vi "GRBLCore.vi"(4 "SecondaryDataFeed":refnum<queue>, 5 "NumOfAxis":i32=3, 6 "MotorDisabled":refnum<vi>, 7 "Simulation":bool, 8 "error in":errorcluster, 9 "Serial Configuration":T2={"Baud Rate"=115200, "Parity"=0, "Data Bits"=8, "Stop Bits"=10, "Flow Control"=0} {"Flow Control" items=["None", "XON/XOFF", "RTS/CTS", "XON/XOFF & RTS/CTS", "DTR/DSR", "XON/XOFF & DTR/DSR"]; "Stop Bits" items=["1.0"=10, "1.5"=15, "2.0"=20]; "Data Bits" items=["7"=7, "8"=8]; "Parity" items=["None", "Odd", "Even", "Mark", "Space"]; "Baud Rate" items=["300"=300, "600"=600, "1200"=1200, "2400"=2400, "4800"=4800, "9600"=9600, "19200"=19200]}, 10 "CommPort":refnum<visa-resource-name>, 11 "ControlQueue in":refnum<queue>) -> (0 "error out":errorcluster, 3 "queue out":refnum<queue>)   [LabVIEW 2014, in "GRBLMotionCore.lvlib"]
uses:
  <instrlib>/GRBL/GRBLMotionCore.lvlib
  <instrlib>/GRBL/Public/Data/GRBL_State.ctl
  <instrlib>/GenericMotionCore/Public/SecondaryDataFeed.ctl
  <instrlib>/GRBL/Public/Data/GRBL_Data.ctl
  <vilib>/Utility/error.llb/DialogType.ctl
  <userlib>/Utility/ErrorLog_lib.lvlib
  <instrlib>/GenericMotionCore/GenericMotionCore.lvlib
panel:
  out "State(Blocking)":T1(ring)
  out "Blokcing Loop cts":i32
  in  "Track Input":bool
  in  "SoftReset":bool caption="Go"
  out "Com failure#":i32
  in  "Go_MoveRel":bool caption="Go"
  out "tick_start":u32
  out "tick_stop":u32
  out "Returned_String":string
  out "refresh rate":i32
  out "resfresh counter":i32
  in  "MotorDisabled":bool caption="Go"
  in  "Home":bool caption="Go"
  in  "StepWidth":dbl(ring)=0.2 items=["0.2 um"=0.0002, "0.001 mm"=0.001, "0.002 mm"=0.002, "0.005 mm "=0.005, "0.01 mm"=0.01, "0.02 mm"=0.02, "0.05 mm"=0.05, "0.1 mm"=0.1, "0.2 mm"=0.2, "1 mm"=1.0]
  in  "Z-":bool
  in  "Z+":bool
  in  "X+":bool
  in  "X-":bool
  in  "Y-":bool
  in  "Y+":bool
  in  "ClearErr":bool caption="Go"
  in  "STOP":bool caption="Go"
  in  "Quit":bool caption="Go"
  out "Instrument Driver Revision":string
  out "Instrument Firmware Revision":string
  in  "SetPosition":dbl[](array[numeric])=[1.0, 1.0, 1.0] caption="Position" format="%.4f"
  in  "SetVelocity":dbl[](array[numeric])=[1.0] caption="Velocity (mm/s)"
  in  "SetAcceleration":dbl[](array[numeric])=[50.0] caption="Acceleration"
  in  "Go":bool
  out "Moving":bool
  out "Acceleration":dbl[](array[numeric])
  out "Velocity":dbl[](array[numeric])
  out "Position":dbl[](array[numeric])
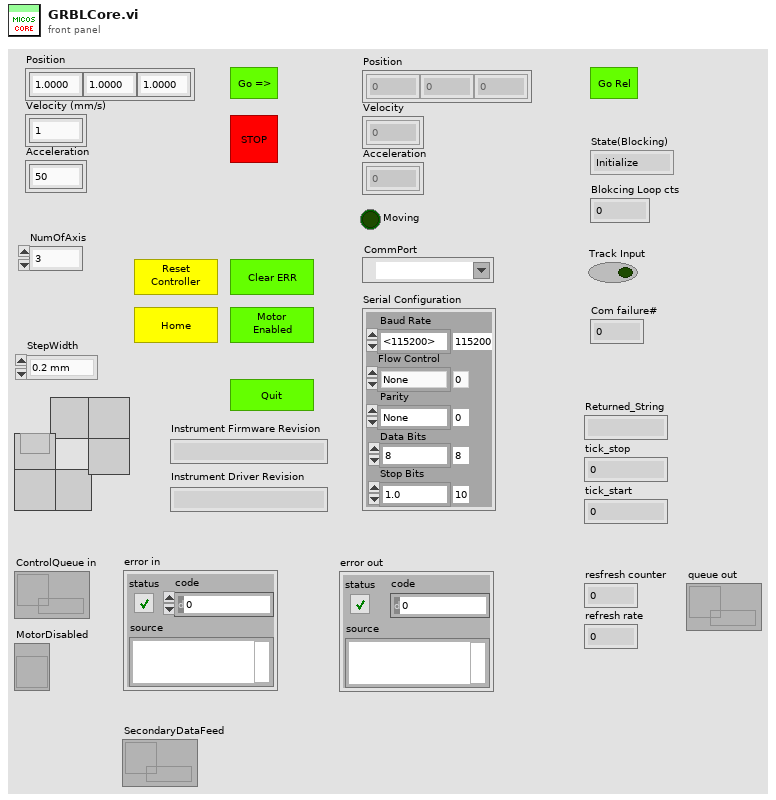
[diagram p1: front panel]
types:
  T1 = enum16{"Initialize", "SetDefaultConfig", "Close", "Quit", "Identify", "MoveAbs", "MoveAbs_all", "MoveRel", "MoveRel_all", "STOP", "Origin/Home", "WaitStop", "QueryStatus", "UpdateXPos", "UpdateAll", "SetVelocity", "SetAcceleration", "ClearErr", "LogMessage", "MotorEnable(1)", "EnableAxis", "JoyStick", "GetVelocity", "GetAcceleration", "SendCmd", "SetSoftLimits", "Beep", "_SettingReturn", "SoftReset"}
  T2 = cluster{"Baud Rate":u32, "Parity":u16, "Data Bits":u16, "Stop Bits":u16, "Flow Control":u16}
  T3 = cluster{"CommPort":refnum<vi>, "Serial Configuration":refnum<vi>, "SetPosition":refnum<vi>, "SetAcceleration":refnum<vi>, "SetVelocity":refnum<vi>, "StepWidth":refnum<vi>, "WaitStopReturn_Queue":refnum<queue>}
  T4 = typedef "GRBLMotionCore.lvlib/GRBL_State.ctl" = cluster{"State":enum16{"Initialize", "SetDefaultConfig", "Close", "Quit", "Identify", "MoveAbs", "MoveAbs_all", "MoveRel", "MoveRel_all", "STOP", "Origin/Home", "WaitStop", "QueryStatus", "UpdateXPos", "UpdateAll", "SetVelocity", "SetAcceleration", "ClearErr", "LogMessage", "MotorEnable(1)", "EnableAxis", "JoyStick", "GetVelocity", "GetAcceleration", "SendCmd", "SetSoftLimits", "Beep", "_SettingReturn", "SoftReset"}, "Params.":variant}
  T5 = typedef "GRBLMotionCore.lvlib/GRBL_Data.ctl" = cluster{"Position":dbl[], "Velocity":dbl[], "Acceleration":dbl[], "Moving":bool, "Simulation":bool, "tickcount_mov":u32, "tickcount_pos":u32, "NumOfAxis":i32, "Initialized":bool, "CommPort":refnum<visa-resource-name>, "Range":dbl[][], "Serial Configuration":cluster{"Baud Rate":u32, "Parity":u16, "Data Bits":u16, "Stop Bits":u16, "Flow Control":u16}, "MotorDisabled":refnum<vi>}
  T6 = typedef "StepWidthSelector.ctl" = dbl
  T7 = typedef "GenericMotionCore.lvlib/SecondaryDataFeed.ctl" = cluster{"tickcount":u32, "SecondaryData":dbl[]}
  T8 = enum16{"Initialize", "SetDefaultConfig", "Close", "Quit", "Identify", "MoveAbs", "MoveAbs_all", "MoveRel", "MoveRel_all", "STOP", "Origin/Home", "WaitStop", "QueryStatus", "UpdateXPos", "UpdateAll", "SetVelocity", "SetAcceleration", "ClearErr", "LogMessage", "MotorEnable(1)", "EnableAxis", "JoyStick", "GetVelocity", "GetAcceleration", "SendCmd", "SetSoftLimits", "Beep", "_SettingReturn"}
  T9 = enum16{"Initialize", "SetDefaultConfig", "Close", "Quit", "Identify", "MoveAbs", "MoveAbs_all", "MoveRel", "MoveRel_all", "STOP", "Origin/Home", "WaitStop", "QueryStatus", "UpdateXPos", "UpdateAll", "SetVelocity", "SetAcceleration", "ClearErr", "LogMessage", "MotorEnable(1)", "EnableAxis", "JoyStick", "GetVelocity", "GetAcceleration", "SendCmd", "SetSoftLimits", "Beep", "_SettingReturn"}[]
  T10 = typedef "DialogType.ctl" = u16
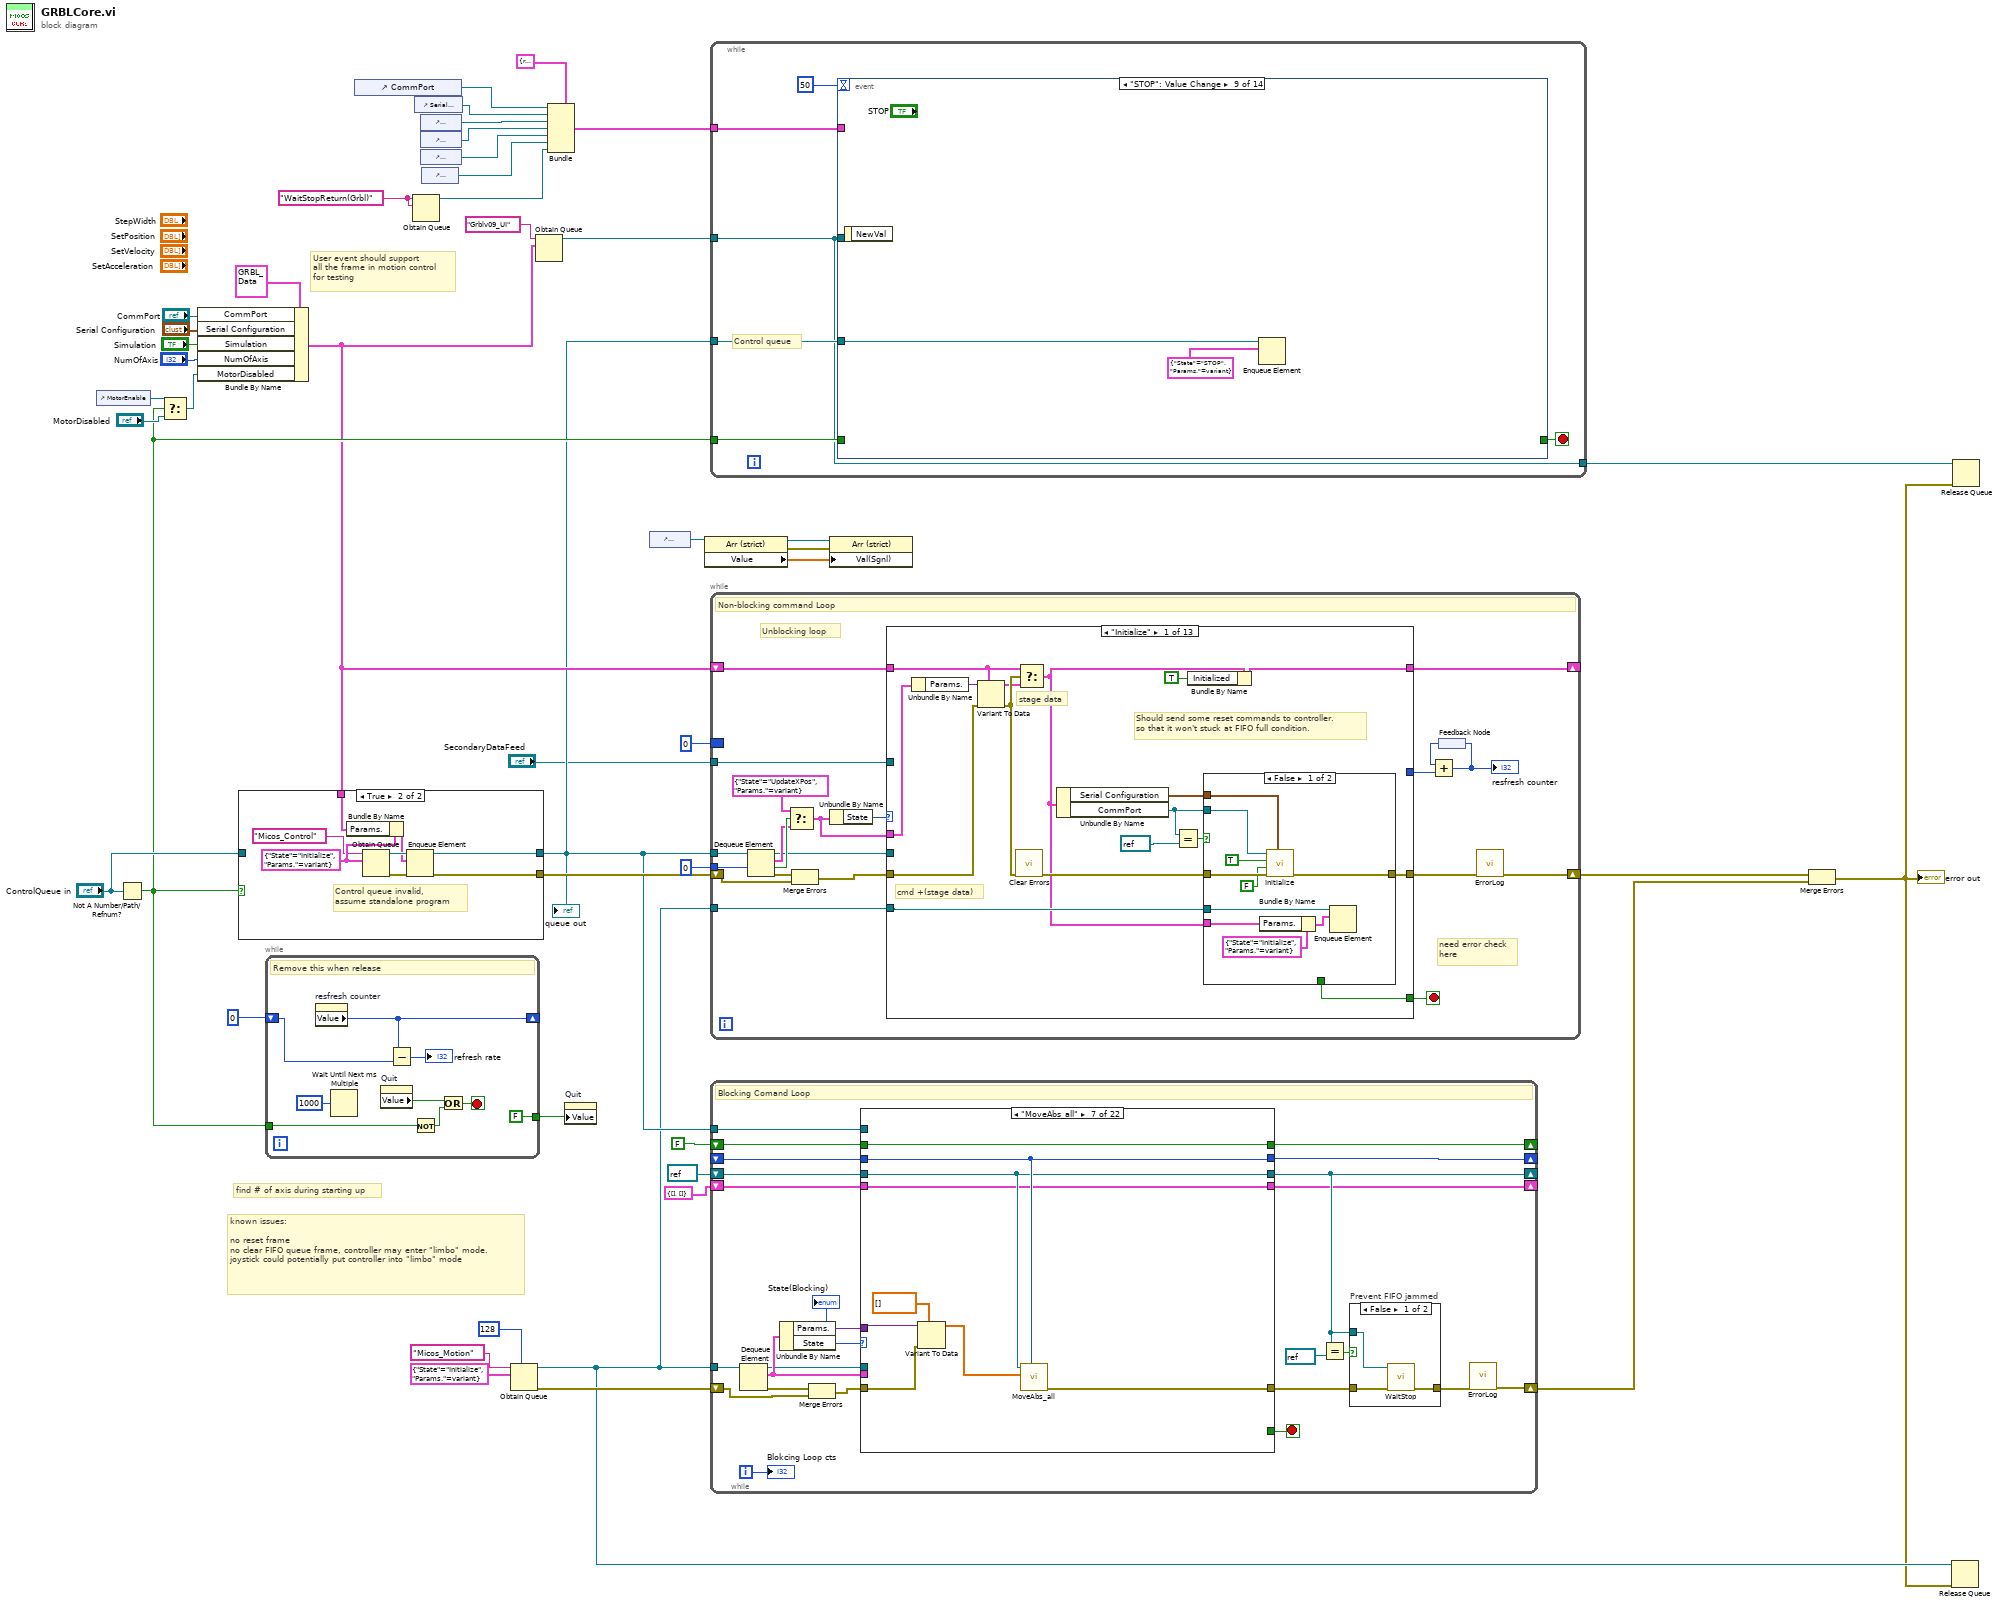
[diagram p0: block diagram]
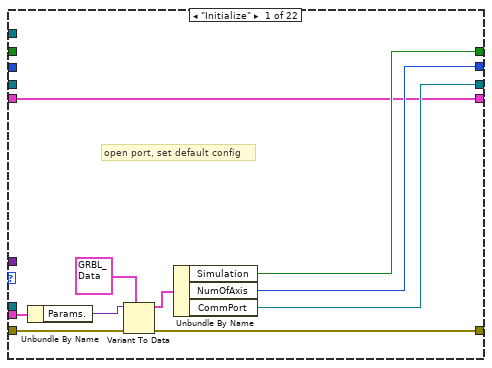
[diagram p3: hidden frame]
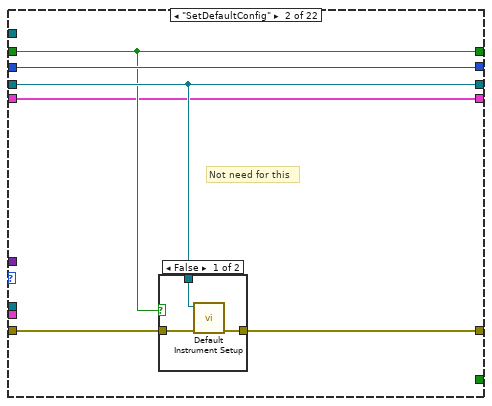
[diagram p4: hidden frame]
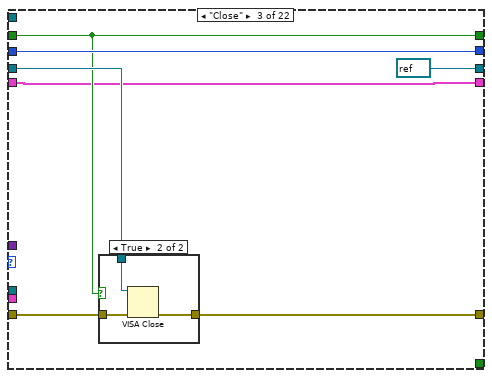
[diagram p6: hidden frame]
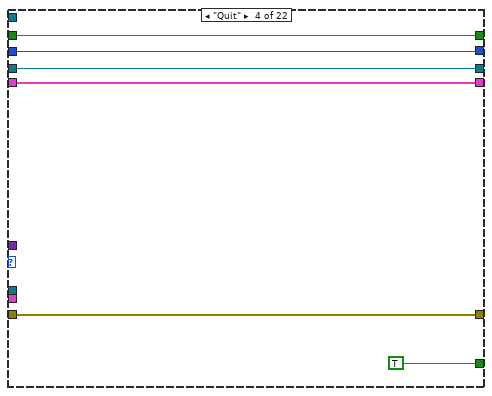
[diagram p8: hidden frame]
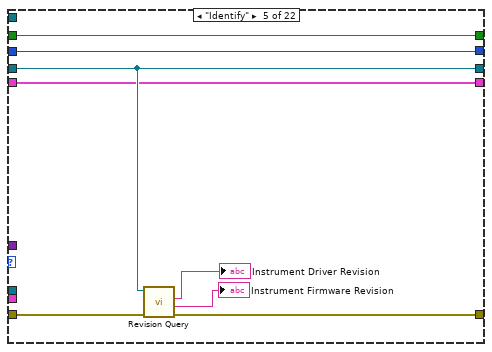
[diagram p9: hidden frame]
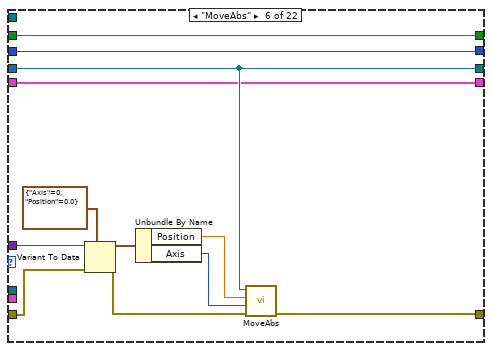
[diagram p10: hidden frame]
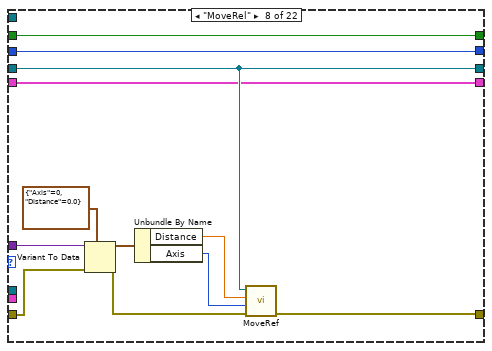
[diagram p11: hidden frame]
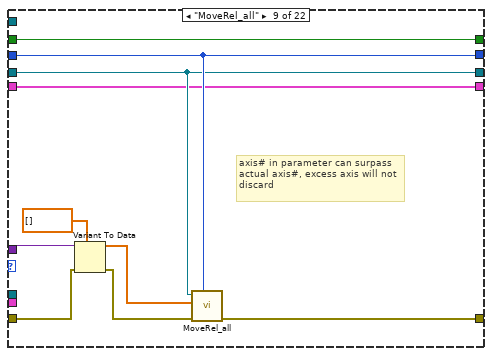
[diagram p12: hidden frame]
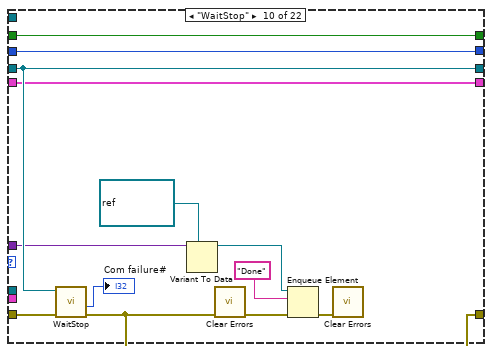
[diagram p13: hidden frame]
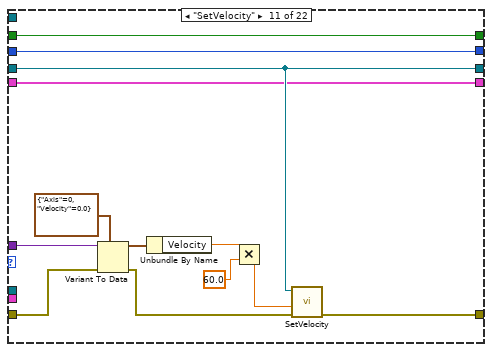
[diagram p14: hidden frame]
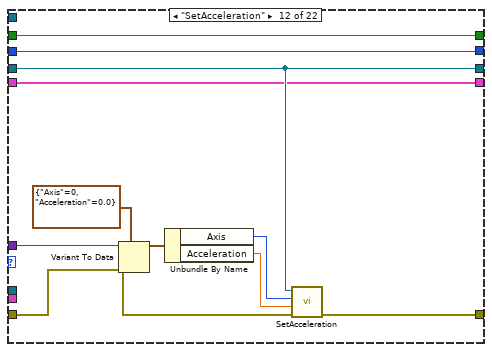
[diagram p15: hidden frame]
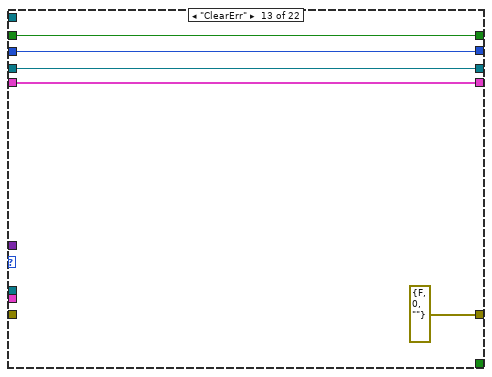
[diagram p16: hidden frame]
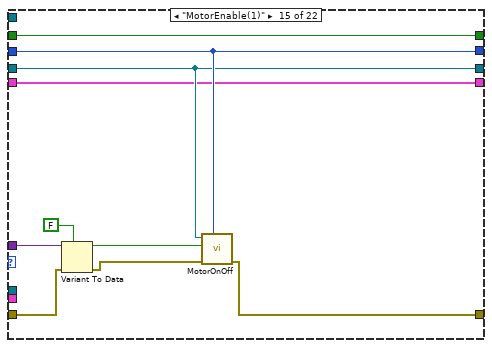
[diagram p18: hidden frame]
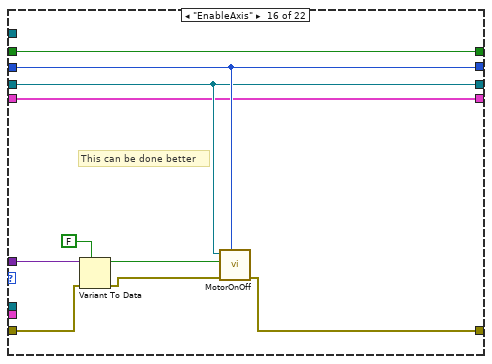
[diagram p19: hidden frame]
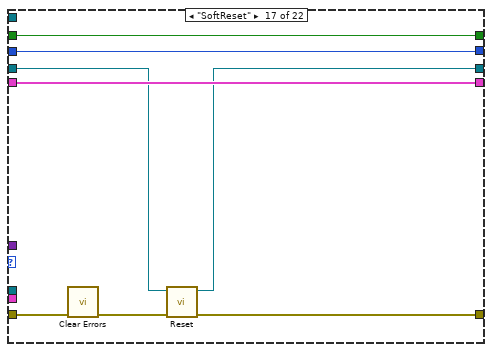
[diagram p20: hidden frame]
diagram:
  w21 = "WaitStopReturn(Grbl)" ("name (unnamed)")
  # "known issues:\n\nno reset frame\nno clear FIFO queue frame, controller may enter \"limbo\" mode. \njoystick could potentially put controller into \"limbo\" mode"
  # "find # of axis during starting up"
  # "User event should support \nall the frame in motion control\nfor testing"
  n1 = control-ref of="MotorEnable"() -> (w28:refnum<vi>)
  n2 = Not A Number/Path/Refnum?(number/path/refnum="ControlQueue in") -> (NaN/Path/Refnum?=w23:bool)
  n3 = Select(t=w28, s=w23, f="MotorDisabled") -> (s? t:f=w26:refnum<vi>)
  n4 = Bundle By Name(cluster=T5 {"Position"=[], "Velocity"=[], "Acceleration"=[], "Moving"=FALSE, "Simulation"=FALSE, "tickcount_mov"=0, "tickcount_pos"=0, "NumOfAxis"=0, "Initialized"=FALSE, "CommPort"="", "Range"=[], "Serial Configuration"={"Baud Rate"=0, "Parity"=0, "Data Bits"=0, "Stop Bits"=0, "Flow Control"=0}, "MotorDisabled"=refnum}, "CommPort"="CommPort", "Serial Configuration"="Serial Configuration", "Simulation"="Simulation", "NumOfAxis"="NumOfAxis", "MotorDisabled"=w26) -> (w22:T5)
  n5 = case shown="True" w23 {
    tunnel: [w48 w54] -> w17
    tunnel: ["error in" w53] -> w46
    tunnel: "ControlQueue in" -> [w48 _]
    tunnel: w22 -> [_ w50]
    frame False {
    }
    frame True {
      w55 = T4 {"State"=enum."Initialize", "Params."=variant}
      # "Control queue invalid, \nassume standalone program"
      n6 = Bundle By Name(cluster=w55, "Params."=w50) -> (w51:T4)
      n7 = Obtain Queue(name (unnamed)="Micos_Control", element data type=w55) -> (queue out=w56:refnum<queue>, error out=w52:errorcluster)  [unwired: 3 in, 1 out]
      n8 = Enqueue Element(queue=w56, element=w51, error in (no error)=w52) -> (queue out=w54:refnum<queue>, error out=w53:errorcluster)  [unwired: 1 in, 1 out]
    }
  }
  "queue out" <- w17
  n9 = while {
    shift-right: [w62] -> _
    shift-left: 0 ("resfresh counter") -> [w65]
    tunnel: w23 -> [w59]
    tunnel: [FALSE ("Quit")] -> w5
    stop <- w60 stop-if-true
    # "Remove this when release"
    n10 = property on="resfresh counter" class="DigNum (strict)"() -> ("Value"=w62:i32)  [unwired: 2 in, 2 out]
    n11 = Wait Until Next ms Multiple(millisecond multiple=u32 1000) -> ()  [unwired: 1 out]
    n12 = property on="Quit" class="Bool (strict)"() -> ("Value"=w63:bool)  [unwired: 2 in, 2 out]
    n13 = Subtract(x=w62, y=w65) -> (x-y=→"refresh rate":i32)
    n14 = Not(x=w59) -> (.not. x?=w58:bool)
    n15 = Or(x=w63, y=w58) -> (x .or. y?=w60:bool)
  }
  n16 = control-ref of="CommPort"() -> (w38:refnum<vi>)
  n17 = Obtain Queue(name (unnamed)=w21, element data type=w21) -> (queue out=w20:refnum<queue>)  [unwired: 3 in, 2 out]
  n18 = control-ref of="Serial Configuration"() -> (w39:refnum<vi>)
  n19 = control-ref of="SetPosition"() -> (w37:refnum<vi>)
  n20 = control-ref of="SetAcceleration"() -> (w36:refnum<vi>)
  n21 = control-ref of="SetVelocity"() -> (w35:refnum<vi>)
  n22 = control-ref of="StepWidth"() -> (w29:refnum<vi>)
  n23 = Obtain Queue(max queue size (-1, unlimited)=128, name (unnamed)="Micos_Motion", element data type=T4 {"State"=enum."Initialize", "Params."=variant}) -> (queue out=w15:refnum<queue>, error out=w43:errorcluster)  [unwired: 2 in, 1 out]
  n24 = Obtain Queue(name (unnamed)="Grblv09_UI", element data type=w22) -> (queue out=w18:refnum<queue>)  [unwired: 3 in, 2 out]
  n25 = Bundle(cluster=T3 {"CommPort"=refnum, "Serial Configuration"=refnum, "SetPosition"=refnum, "SetAcceleration"=refnum, "SetVelocity"=refnum, "StepWidth"=refnum, "WaitStopReturn_Queue"=refnum}, "CommPort"=w38, "Serial Configuration"=w39, "SetPosition"=w37, "SetAcceleration"=w36, "SetVelocity"=w35, "StepWidth"=w29, "WaitStopReturn_Queue"=w20) -> (w34:T3)
  n26 = property on="Quit" class="Bool (strict)"("Value"=w5) -> ()  [unwired: 2 in, 2 out]
  n27 = control-ref of="SetVelocity"() -> (w1:refnum<vi>)
  n28 = property class="Arr (strict)"(reference=w1) -> (reference out=w2:refnum<vi>, error out=w3:errorcluster, "Value"=w4:dbl[])  [unwired: 1 in]
  n29 = while {
    tunnel: w17 -> [w67]
    tunnel: w23 -> [w70]
    tunnel: w18 -> [w66]
    tunnel: w34 -> [w68]
    tunnel: [w66] -> w16
    stop <- w71 stop-if-true
    # "Control queue"
    n30 = event shown="[8] \"STOP\": Value Change" {
      selector: _ -> [_ _ _ _ _ _ _ _ _ _ _ _ _ _]
      dyn-events: _ -> [_ _ _ _ _ _ _ _ _ _ _ _ _ _]
      timeout: 50 -> [_ _ _ _ _ _ _ _ _ _ _ _ _ _]
      tunnel: [w74 _ _ _ _ _ _ _ _ _ _ TRUE _ _] -> w71
      tunnel: w70 -> [w87 _ _ _ _ _ _ _ _ _ _ _ _ _]
      tunnel: w67 -> [w86 w106 w117 w126 w135 w146 _ w180 w186 w188 w193 w196 w199 w201]
      tunnel: w66 -> [w79 _ _ _ _ _ _ _ _ _ _ _ _ _]
      tunnel: w68 -> [w78 w105 w116 _ _ _ w158 w179 _ _ _ _ _ _]
      event Timeout {
        # "Send return queue ref"
        n31 = event-data() -> ()  [unwired: 1 in, 1 out]
        n32 = Unbundle By Name(w78) -> ("WaitStopReturn_Queue"=w73:refnum<queue>)
        n33 = Not(x=w87) -> (.not. x?=w74:bool)
        n34 = Bundle By Name(cluster=T4 {"State"=enum."QueryStatus", "Params."=variant} ("element"), "Params."=w79) -> (w84:T4)
        n35 = Enqueue Element(queue=w86, element=w84) -> (error out=w82:errorcluster)  [unwired: 2 in, 2 out]
        n36 = Dequeue Element(queue=w79, timeout in ms (-1)=1000, error in (no error)=w82) -> (element=w80:T5, timed out?=w81:bool)  [unwired: 2 out]
        n37 = case shown="False" w81 {
          tunnel: w80 -> [w95 _]
          frame False {
            n38 = Unbundle By Name(w95) -> ("Position"=→"Position":dbl[], "Velocity"=→"Velocity":dbl[], "Acceleration"=→"Acceleration":dbl[], "Moving"=→"Moving":bool)
          }
          frame True {
          }
        }
        n39 = Dequeue Element(queue=w73, timeout in ms (-1)=0) -> (queue out=w72:refnum<queue>, element=w77:string, timed out?=w76:bool)  [unwired: 1 in, 1 out]
        n40 = case "Non-blocking WaitStop in UI for testing" shown="False" w76 {
          tunnel: w77 -> [w89 _]
          frame False {
            # "Non-blocking Wait for testing"
            n41 = Tick Count (ms)() -> (millisecond timer value=→"tick_stop":u32)
            "Returned_String" <- w89
          }
          frame True {
          }
        }
        n42 = case "Release feedback queue if no UI" shown="True" w74 {
          tunnel: w72 -> [_ w88]
          frame False {
          }
          frame True {
            n43 = Release Queue(queue=w88) -> ()  [unwired: 2 in, 3 out]
          }
        }
      }
      event "Go": Value Change {
        n44 = Unbundle By Name(w105) -> ("WaitStopReturn_Queue"=w100:refnum<queue>, "SetPosition"=w104:refnum<vi>)
        n45 = event-data() -> ()  [unwired: 1 in, 1 out]
        n46 = flat-sequence {
          tunnel: w106 -> [w113]
          tunnel: w103 -> [w110]
          tunnel: [w109] -> w102
          tunnel: [w108] -> w101
          frame #0 {
            n47 = Tick Count (ms)() -> (millisecond timer value=→"tick_start":u32)
            n48 = Bundle By Name(cluster=T4 {"State"=enum."MoveAbs_all", "Params."=variant} ("element"), "Params."=w110) -> (w111:T4)
            n49 = Enqueue Element(queue=w113, element=w111) -> (queue out=w109:refnum<queue>, error out=w108:errorcluster)  [unwired: 2 in, 1 out]
          }
        }
        n50 = property class="Arr (strict)"(reference=w104) -> ("Value"=w103:dbl[])  [unwired: 1 in, 2 out]
        n51 = local write "Returned_String"("Done" ("Returned_String")) -> ()
        n52 = local write "tick_stop"(u32 0 ("tick_stop")) -> ()
        n53 = Bundle By Name(cluster=T4 {"State"=enum."WaitStop", "Params."=variant} ("element"), "Params."=w100) -> (w97:T4)
        n54 = Enqueue Element(queue=w102, element=w97, error in (no error)=w101) -> ()  [unwired: 1 in, 3 out]
      }
      event "Go_MoveRel": Value Change {
        n55 = event-data() -> ()  [unwired: 1 in, 1 out]
        n56 = Unbundle By Name(w116) -> ("SetPosition"=w115:refnum<vi>)
        n57 = flat-sequence {
          tunnel: w117 -> [w123]
          tunnel: w114 -> [w120]
          tunnel: [w119] -> _
          tunnel: [w118] -> _
          frame #0 {
            n58 = Bundle By Name(cluster=T4 {"State"=enum."MoveRel_all", "Params."=variant} ("element"), "Params."=w120) -> (w121:T4)
            n59 = Enqueue Element(queue=w123, element=w121) -> (queue out=w119:refnum<queue>, error out=w118:errorcluster)  [unwired: 2 in, 1 out]
          }
        }
        n60 = property class="Arr (strict)"(reference=w115) -> ("Value"=w114:dbl[])  [unwired: 1 in, 2 out]
      }
      event "SetPosition": Value Change {
        n61 = event-data() -> ("NewVal"=w125:dbl[])  [unwired: 1 in]
        n62 = case shown="True" "Track Input" {
          tunnel: w126 -> [_ w130]
          tunnel: w125 -> [_ w127]
          frame False {
          }
          frame True {
            n63 = Bundle By Name(cluster=T4 {"State"=enum."MoveAbs_all", "Params."=variant} ("element"), "Params."=w127) -> (w128:T4)
            n64 = Enqueue Element(queue=w130, element=w128) -> ()  [unwired: 2 in, 3 out]
          }
        }
      }
      event "SetVelocity": Value Change {
        n65 = event-data() -> ("NewVal"=w134:dbl[])  [unwired: 1 in]
        n66 = for {
          N: 1 -> [_]
          tunnel: w134 -> [w138] mode=indexing
          shift-right: [w137] -> w133
          shift-left: w135 -> [w137]
          i -> [w143]
          n67 = Increment(x=w143) -> (x+1=w142:i32)
          n68 = Bundle By Name(cluster=cluster{"Axis":i32, "Velocity":dbl} {"Axis"=0, "Velocity"=0.0}, "Velocity"=w138, "Axis"=w142) -> (w139:cluster{"Axis":i32, "Velocity":dbl})
          n69 = Bundle By Name(cluster=T4 {"State"=enum."SetVelocity", "Params."=variant} ("element"), "Params."=w139) -> (w141:T4)
          n70 = Enqueue Element(queue=w137, element=w141) -> ()  [unwired: 2 in, 3 out]
        }
        n71 = Enqueue Element(queue=w133, element=T4 {"State"=enum."GetVelocity", "Params."=variant}) -> ()  [unwired: 2 in, 3 out]
      }
      event "SetAcceleration": Value Change {
        n72 = event-data() -> ("NewVal"=w147:dbl[])  [unwired: 1 in]
        n73 = for {
          tunnel: w147 -> [w149] mode=indexing
          shift-right: [w148] -> w144
          shift-left: w146 -> [w148]
          i -> [w155]
          n74 = Increment(x=w155) -> (x+1=w153:i32)
          n75 = Bundle By Name(cluster=cluster{"Axis":i32, "Acceleration":dbl} {"Axis"=0, "Acceleration"=0.0}, "Acceleration"=w149, "Axis"=w153) -> (w150:cluster{"Axis":i32, "Acceleration":dbl})
          n76 = Bundle By Name(cluster=T4 {"State"=enum."SetAcceleration", "Params."=variant} ("element"), "Params."=w150) -> (w152:T4)
          n77 = Enqueue Element(queue=w148, element=w152) -> ()  [unwired: 2 in, 3 out]
        }
        n78 = Enqueue Element(queue=w144, element=T4 {"State"=enum."GetAcceleration", "Params."=variant}) -> ()  [unwired: 2 in, 3 out]
      }
      event "Position": Mouse Down {
        n79 = event-data() -> ("CtlRef"=w157:refnum<vi>, "Mods.Double Click"=w156:bool)  [unwired: 1 in]
        n80 = case shown="True" w156 {
          tunnel: w158 -> [_ w162]
          tunnel: w157 -> [_ w160]
          frame False {
          }
          frame True {
            n81 = Unbundle By Name(w162) -> ("SetPosition"=w161:refnum<vi>)
            n82 = property class="Arr (strict)"(reference=w160) -> ("Value"=w159:dbl[])  [unwired: 1 in, 2 out]
            n83 = property class="Arr (strict)"(reference=w161, "Value"=w159) -> ()  [unwired: 1 in, 2 out]
          }
        }
      }
      event "X+", "X-", "Y+", "Y-", "Z+", "Z-": Value Change {
        n84 = event-data() -> ()  [unwired: 1 in, 1 out]
        n85 = Unbundle By Name(w179) -> ("StepWidth"=w178:refnum<vi>)
        n86 = property class="Ring (strict)"(reference=w178) -> ("Value"=w170:T6)  [unwired: 1 in, 2 out]
        n87 = Build Array("X+", "X-", "Y+", "Y-", "Z+", "Z-") -> (w177:bool[])
        n88 = Search 1D Array(1D array=w177, element=TRUE) -> (index of element=w174:i32)  [unwired: 1 in]
        n89 = Index Array(array=dbl[] [1.0, -1.0, 1.0, -1.0, 1.0, -1.0], index=w174) -> (element=w173:dbl)
        n90 = Index Array(array=i32[] [1, 1, 2, 2, 3, 3], index=w174) -> (element=w169:i32)
        n91 = Multiply(x=w170, y=w173) -> (x*y=w171:T6)
        n92 = Bundle By Name(cluster=cluster{"Axis":i32, "Position":dbl} {"Axis"=0, "Position"=0.0}, "Position"=w171, "Axis"=w169) -> (w181:cluster{"Axis":i32, "Position":dbl})
        n93 = Bundle By Name(cluster=T4 {"State"=enum."MoveRel", "Params."=variant} ("element"), "Params."=w181) -> (w183:T4)
        n94 = Enqueue Element(queue=w180, element=w183) -> ()  [unwired: 2 in, 3 out]
      }
      event "STOP": Value Change {
        n95 = event-data() -> ()  [unwired: 1 in, 1 out]
        n96 = Enqueue Element(queue=w186, element=T4 {"State"=enum."STOP", "Params."=variant}) -> ()  [unwired: 2 in, 3 out]
      }
      event "Home": Value Change {
        n97 = event-data() -> ()  [unwired: 1 in, 1 out]
        n98 = Enqueue Element(queue=w188, element=T4 {"State"=enum."Origin/Home", "Params."=variant}) -> ()  [unwired: 2 in, 3 out]
      }
      event "MotorDisabled": Value Change {
        n99 = event-data() -> ()  [unwired: 1 in, 1 out]
        n100 = Not(x="MotorDisabled") -> (.not. x?=w189:bool)
        n101 = Bundle By Name(cluster=T4 {"State"=enum."MotorEnable(1)", "Params."=variant} ("element"), "Params."=w189) -> (w191:T4)
        n102 = Enqueue Element(queue=w193, element=w191) -> ()  [unwired: 2 in, 3 out]
      }
      event "Quit": Value Change {
        n103 = event-data() -> ()  [unwired: 1 in, 1 out]
        n104 = disable-structure shown="Disabled" {
          frame Disabled {
            n105 = property on="Quit" class="Bool (strict)"("Value"=FALSE ("Quit")) -> ()  [unwired: 2 in, 2 out]
          }
          frame Enabled {
          }
        }
        n106 = Enqueue Element(queue=w196, element=T4 {"State"=enum."Quit", "Params."=variant}) -> ()  [unwired: 2 in, 3 out]
      }
      event "ClearErr": Value Change {
        n107 = event-data() -> ()  [unwired: 1 in, 1 out]
        n108 = Enqueue Element(queue=w199, element=T4 {"State"=enum."ClearErr", "Params."=variant}) -> ()  [unwired: 2 in, 3 out]
      }
      event "SoftReset": Value Change {
        n109 = event-data() -> ()  [unwired: 1 in, 1 out]
        n110 = Enqueue Element(queue=w201, element=T4 {"State"=enum."SoftReset", "Params."=variant}) -> ()  [unwired: 2 in, 3 out]
      }
    }
  }
  n111 = while {
    tunnel: w17 -> [w212]
    shift-right: [w222] -> _
    shift-left: w22 -> [w221]
    tunnel: w15 -> [w219]
    shift-right: [w203] -> w8
    shift-left: w46 -> [w208]
    tunnel: 0 ("f") -> [w210]
    border: 0 -> [_]
    tunnel: "SecondaryDataFeed" -> [w202]
    stop <- w220 stop-if-true
    # "Unblocking loop"
    # "need error check\nhere"
    # "Non-blocking command Loop"
    n112 = Dequeue Element(queue=w212, timeout in ms (-1)=w210) -> (queue out=w213:refnum<queue>, element=w215:T4, timed out?=w217:bool, error out=w218:errorcluster)  [unwired: 1 in]
    n113 = Select(t=T4 {"State"=enum."UpdateXPos", "Params."=variant} ("element"), s=w217, f=w215) -> (s? t:f=w214:T4)
    n114 = Merge Errors(w218, w208) -> (w209:errorcluster)
    n115 = Unbundle By Name(w214) -> ("State"=w211:T1)
    n116 = case shown="\"Initialize\"" w211 {
      tunnel: w214 -> [w230 w262 _ _ w317 _ _ _ _ w429 w448 w460 w473]
      tunnel: [w239 w259 w279 w303 w313 w322 w345 w387 w425 w434 w451 w458 w475] -> w222
      tunnel: w221 -> [w233 w257 w279 w303 w313 w322 w343 w385 w425 w434 w451 w461 w475]
      tunnel: [w229 _ TRUE _ _ _ _ _ _ _ _ _ _] -> w220
      tunnel: w219 -> [w224 w263 w282 w302 _ _ _ w374 _ w433 w450 _ _]
      tunnel: [w232 w260 w284 w298 w315 w320 w336 w377 errorcluster {"status"=FALSE, "code"=0, "source"=""} ("error out") w426 w447 w452 w476] -> w204
      tunnel: w209 -> [w236 w261 w280 w301 w316 w323 w344 w386 _ w432 w449 w453 _]
      tunnel: w213 -> [_ w255 _ _ _ _ w335 _ _ w430 _ _ w468]
      tunnel: [_ _ _ _ _ _ 1 1 _ _ _ _ _] -> w207
      tunnel: w202 -> [_ _ _ _ _ _ w325 w371 _ _ _ _ _]
      frame "Initialize" {
        # "Should send some reset commands to controller. \nso that it won't stuck at FIFO full condition."
        # "cmd +(stage data)"
        # "stage data"
        n117 = Unbundle By Name(w230) -> ("Params."=w237:variant)
        n118 = Variant To Data(error in=w236, type=w233, Variant=w237) -> (data=w234:T5, error out=w235:errorcluster)
        n119 = call <vilib>:"Clear Errors.vi"("error in (no error)"=w235) -> ("error out"=w225:errorcluster)  [unwired: 5 in, 1 out]
        n120 = Select(t=w233, s=w235, f=w234) -> (s? t:f=w223:T5)
        n121 = Unbundle By Name(w223) -> ("Serial Configuration"=w231:T2, "CommPort"=w227:refnum<visa-resource-name>)
        n122 = Equal?(x=w227, y=refnum<visa-resource-name> refnum ("CommPort")) -> (x = y?=w228:bool)
        n123 = Bundle By Name(cluster=w223, "Initialized"=TRUE) -> (w239:T5)
        n124 = case shown="False" w228 {
          tunnel: w225 -> [w249 w252]
          tunnel: [w248 errorcluster {"status"=FALSE, "code"=-5104, "source"="Device unspecifiied,\nSkip execution"} ("error out")] -> w232
          tunnel: w231 -> [w247 _]
          tunnel: w227 -> [w246 _]
          tunnel: [_ w250] -> w229
          tunnel: w224 -> [w241 w254]
          tunnel: w223 -> [w240 _]
          frame False {
            n125 = Bundle By Name(cluster=T4 {"State"=enum."Initialize", "Params."=variant}, "Params."=w240) -> (w243:T4)
            n126 = call <instrlib>:"Initialize.vi"("Serial Configuration"=w247, "error in (no error)"=w249, "Reset (True)"=FALSE, "ID Query (True)"=TRUE, "VISA resource name"=w246) -> ("error out"=w248:errorcluster)  [unwired: 5 in, 1 out]
            n127 = Enqueue Element(queue=w241, element=w243) -> ()  [unwired: 2 in, 3 out]
          }
          frame True {
            w250 = TRUE
            n128 = Enqueue Element(queue=w254, element=T4 {"State"=enum."Quit", "Params."=variant}, error in (no error)=w252) -> ()  [unwired: 1 in, 3 out]
            n129 = property on="Quit" class="Bool (strict)"("Val(Sgnl)"=w250) -> ()  [unwired: 2 in, 2 out]
          }
        }
      }
      frame "Close" {
        n130 = Unbundle By Name(w257) -> ("Moving"=w256:bool)
        n131 = case shown="True" w256 {
          tunnel: w263 -> [w267 _]
          tunnel: w262 -> [w266 w268]
          tunnel: w261 -> [w265 w272]
          tunnel: [w264 w269] -> w260
          tunnel: w255 -> [_ w277]
          frame False {
            n132 = Enqueue Element "Imply \"Close\""(queue=w267, element=w266, error in (no error)=w265) -> (error out=w264:errorcluster)  [unwired: 1 in, 2 out]
          }
          frame True {
            n133 = Enqueue Element At Opposite End "Implied \"Close\""(queue=w277, element=w268, error in (no error)=w272) -> (queue out=w276:refnum<queue>, error out=w271:errorcluster)  [unwired: 1 in, 1 out]
            n134 = Enqueue Element At Opposite End(queue=w276, element=T4 {"State"=enum."UpdateAll", "Params."=variant}, error in (no error)=w271) -> (queue out=w275:refnum<queue>, error out=w270:errorcluster)  [unwired: 1 in, 1 out]
            n135 = Enqueue Element At Opposite End(queue=w275, element=T4 {"State"=enum."STOP", "Params."=variant}, error in (no error)=w270) -> (error out=w269:errorcluster)  [unwired: 1 in, 2 out]
          }
        }
        n136 = Bundle By Name(cluster=w257, "Initialized"=FALSE) -> (w259:T5)
      }
      frame "Quit" {
        n137 = Unbundle By Name(w279) -> ("Initialized"=w278:bool)
        n138 = case shown="True" w278 {
          tunnel: [w288 w292] -> w283
          tunnel: w282 -> [w288 w291]
          tunnel: [w287 w290] -> w281
          tunnel: w280 -> [w287 w289]
          frame False {
          }
          frame True {
            n139 = Enqueue Element(queue=w291, element=T4 {"State"=enum."Close", "Params."=variant}, error in (no error)=w289) -> (queue out=w292:refnum<queue>, error out=w290:errorcluster)  [unwired: 1 in, 1 out]
          }
        }
        n140 = Enqueue Element(queue=w283, element=T4 {"State"=enum."Quit", "Params."=variant}, error in (no error)=w281) -> (error out=w284:errorcluster)  [unwired: 1 in, 2 out]
      }
      frame "STOP" {
        w294 = T9 [enum."WaitStop", enum."UpdateAll", enum."Close", enum."Quit", enum."SetVelocity"] items=["Initialize", "SetDefaultConfig", "Close", "Quit", "Identify", "MoveAbs", "MoveAbs_all", "MoveRel", "MoveRel_all", "STOP", "Origin/Home", "WaitStop", "QueryStatus", "UpdateXPos", "UpdateAll", "SetVelocity", "SetAcceleration", "ClearErr", "LogMessage", "MotorEnable(1)", "EnableAxis", "JoyStick", "GetVelocity", "GetAcceleration", "SendCmd", "SetSoftLimits", "Beep", "_SettingReturn"]
        # "should not dump wait for stop!!"
        # "send stop to controller, update"
        n141 = Unbundle By Name(w303) -> ("CommPort"=w300:refnum<visa-resource-name>)
        n142 = Flush Queue(queue=w302, error in (no error)=w301) -> (queue out=w295:refnum<queue>, remaining elements=w296:T4[], error out=w299:errorcluster)
        n143 = VISA Write(VISA resource name=w300, write buffer="!\r\n" ("Substring"), error in (no error)=w299) -> (error out=w298:errorcluster)  [unwired: 2 out]
        n144 = for {
          tunnel: w296 -> [w309] mode=indexing
          tunnel: w295 -> [w308]
          tunnel: w294 -> [w306]
          n145 = Unbundle By Name(w309) -> ("State"=w307:T1)
          n146 = Equal?(x=w307, y=w306) -> (x = y?=w304:bool[])
          n147 = Or Array Elements(Boolean array=w304) -> (logical OR=w305:bool)
          n148 = case shown="True" w305 {
            tunnel: w309 -> [_ w311]
            tunnel: w308 -> [_ w310]
            frame False {
            }
            frame True {
              n149 = Enqueue Element At Opposite End(queue=w310, element=w311) -> ()  [unwired: 2 in, 3 out]
            }
          }
        }
      }
      frame "QueryStatus" {
        # "return the value to queue"
        n150 = Unbundle By Name(w317) -> ("Params."=w319:variant)
        n151 = Variant To Data(error in=w316, type=refnum<queue> refnum ("queue out"), Variant=w319) -> (data=w314:refnum<queue>, error out=w318:errorcluster)
        n152 = Enqueue Element(queue=w314, element=w313, error in (no error)=w318) -> (error out=w315:errorcluster)  [unwired: 1 in, 2 out]
      }
      frame "Origin/Home" {
        # "The stage won't work, if not calibrated/homed,\nSo calibration has to be in the non-blocking loop\n\nAlso, during calibration, communication stop, causing error"
        n153 = Unbundle By Name(w322) -> ("CommPort"=w321:refnum<visa-resource-name>)
        n154 = call <instrlib>:"OriginSearch.vi"("error in"=w323, "VISA resource"=w321) -> ("error out"=w320:errorcluster)  [unwired: 9 in]
      }
      frame "UpdateXPos" {
        n155 = Unbundle By Name(w343) -> ("NumOfAxis"=w329:i32, "CommPort"=w331:refnum<visa-resource-name>)
        n156 = feedback #1(0) -> (w339:i32)
        n157 = Increment(x=w339) -> (x+1=w340:i32)
        n158 = Quotient & Remainder(x=w340, y=16) -> (x-y*floor(x/y)=w337:i32)  [unwired: 1 out]
        n159 = feedback-in #1(w337) -> ()
        n160 = Equal To 0?(x=w337) -> (x = 0?=w334:bool)
        n161 = call <instrlib>:"Update_xPos.vi"("NumOfAxis"=w329, "error in (no error)"=w344, "VISA resource name"=w331) -> ("error out"=w327:errorcluster, "x_Moving"=w332:bool, "Position"=w330:dbl[], "tickcount_pos"=w342:u32)  [unwired: 5 in]
        n162 = Compound Arithmetic op=OR(invert w332, w334) -> (w333:bool)
        n163 = case shown="No Error" w327 {
          selector: w327 -> [w352 w357]
          tunnel: [w354 w360] -> w345
          tunnel: w343 -> [w353 w360]
          tunnel: w342 -> [w347 _]
          tunnel: w330 -> [w346 _]
          tunnel: [w352 w356] -> w326
          tunnel: w325 -> [w348 _]
          frame No Error {
            n164 = Bundle(cluster=T7 {"tickcount"=0, "SecondaryData"=[]} ("SecondaryDataFeed"), "tickcount"=w347, "SecondaryData"=w346) -> (w349:T7)
            n165 = Bundle By Name(cluster=w353, "tickcount_pos"=w347, "Position"=w346) -> (w354:T5)
            n166 = Lossy Enqueue Element(queue=w348, element=w349) -> (error out=w350:errorcluster)  [unwired: 1 in, 3 out]
            n167 = call <vilib>:"Clear Errors.vi"("error in (no error)"=w350) -> ()  [unwired: 5 in, 2 out]
          }
          frame Error {
            w355 = T10 0 items=["no dialog", "OK message", "continue or stop message", "OK message + warnings", "continue/stop + warnings"] ("type of dialog (OK msg:1)")
            w358 = 1 items=["no exception", "cancel error on match", "set error on match"] ("[exception action] (none:0)")
            n168 = for {
              shift-right: [w364] -> w356
              shift-left: w357 -> [w365]
              tunnel: w358 -> [w363]
              tunnel: i32[] [85, -1073807252, 1, -1073807339] -> [w362] mode=indexing
              tunnel: w355 -> [w361]
              n169 = call <vilib>:"General Error Handler.vi"("type of dialog (OK msg:1)"=w361, "error in (no error)"=w365, "[exception action] (none:0)"=w363, "[exception code]"=w362) -> ("error out"=w364:errorcluster)  [unwired: 7 in, 4 out]
            }
          }
        }
        n170 = Wait Until Next ms Multiple(millisecond multiple=u32 40) -> ()  [unwired: 1 out]
        n171 = case shown="True" w333 {
          tunnel: [w366 w370] -> w336
          tunnel: w335 -> [_ w369]
          tunnel: w326 -> [w366 w367]
          frame False {
          }
          frame True {
            n172 = Enqueue Element At Opposite End(queue=w369, element=T4 {"State"=enum."UpdateAll", "Params."=variant}, error in (no error)=w367) -> (error out=w370:errorcluster)  [unwired: 1 in, 2 out]
          }
        }
      }
      frame "UpdateAll" {
        n173 = Unbundle By Name(w385) -> ("MotorDisabled"=w376:refnum<vi>, "NumOfAxis"=w384:i32, "CommPort"=w383:refnum<visa-resource-name>)
        n174 = call <instrlib>:"Update_all.vi"("# axis"=w384, "error in (no error)"=w386, "VISA resource name"=w383) -> ("error out"=w378:errorcluster, "Moving"=w379:bool, "Currrent postion"=w382:dbl[], "tickcount_pos"=w381:u32, "MotorDisabled"=w372:bool)  [unwired: 4 in]
        n175 = property class="Bool (strict)"(reference=w376, "Blinking"=w372, "Value"=w372) -> (error out=w375:errorcluster)  [unwired: 1 in, 1 out]
        n176 = case shown="No Error" w378 {
          selector: w378 -> [_ w415]
          tunnel: [w406 w418] -> w387
          tunnel: w385 -> [w405 w418]
          tunnel: w382 -> [w389 _]
          tunnel: w381 -> [w390 _]
          tunnel: w379 -> [w403 _]
          tunnel: [_ w414] -> w377
          tunnel: w374 -> [w404 _]
          tunnel: T4[] [{"State"=enum."GetVelocity", "Params."=variant}, {"State"=enum."_SettingReturn", "Params."=variant}] -> [w402 _]
          tunnel: w371 -> [w388 _]
          frame No Error {
            w394 = FALSE  # Bypass  continuous update
            n177 = Tick Count (ms)() -> (millisecond timer value=w400:u32)
            n178 = feedback #2() -> (w396:u32)  [unwired: 1 in]
            n179 = Subtract(x=w400, y=w396) -> (x-y=w399:u32)
            n180 = Greater?(x=u32 1000, y=w399) -> (0:w401:bool)
            n181 = Compound Arithmetic op=OR(w394, w403, w401) -> (w395:bool)
            n182 = Bundle By Name(cluster=w405, "tickcount_pos"=w390, "Position"=w389, "Moving"=w403) -> (w406:T5)
            n183 = case shown="False" w395 {
              tunnel: w404 -> [w409 _]
              tunnel: w402 -> [w408 _]
              tunnel: [w407 w412] -> w397
              tunnel: w396 -> [_ w412]
              frame False {
                n184 = for {
                  tunnel: w409 -> [w411]
                  tunnel: w408 -> [w410] mode=indexing
                  n185 = Enqueue Element(queue=w411, element=w410) -> ()  [unwired: 2 in, 3 out]
                }
                n186 = Tick Count (ms)() -> (millisecond timer value=w407:u32)
              }
              frame True {
              }
            }
            n187 = feedback-in #2(w397) -> ()
            n188 = Bundle(cluster=T7 {"tickcount"=0, "SecondaryData"=[]} ("SecondaryDataFeed"), "tickcount"=w390, "SecondaryData"=w389) -> (w391:T7)
            n189 = Lossy Enqueue Element(queue=w388, element=w391) -> (error out=w392:errorcluster)  [unwired: 1 in, 3 out]
            n190 = call <vilib>:"Clear Errors.vi"("error in (no error)"=w392) -> ()  [unwired: 5 in, 2 out]
          }
          frame Error {
            w413 = T10 0 items=["no dialog", "OK message", "continue or stop message", "OK message + warnings", "continue/stop + warnings"] ("type of dialog (OK msg:1)")
            w417 = 1 items=["no exception", "cancel error on match", "set error on match"] ("[exception action] (none:0)")
            n191 = for {
              shift-right: [w422] -> w414
              shift-left: w415 -> [w423]
              tunnel: w417 -> [w421]
              tunnel: i32[] [85, -1073807252, -1073807339, 1] -> [w420] mode=indexing
              tunnel: w413 -> [w419]
              n192 = call <vilib>:"General Error Handler.vi"("type of dialog (OK msg:1)"=w419, "error in (no error)"=w423, "[exception action] (none:0)"=w421, "[exception code]"=w420) -> ("error out"=w422:errorcluster)  [unwired: 7 in, 4 out]
            }
          }
        }
        n193 = call <vilib>:"Clear Errors.vi"("error in (no error)"=w375) -> ()  [unwired: 5 in, 2 out]
      }
      frame "ClearErr" {
      }
      frame Default {
        # "system does not response \nafter a command is received"
        # "timeout push command back then do update?\n\npreventing blocking"
        n194 = Enqueue Element(queue=w433, element=w429, timeout in ms (-1)=0, error in (no error)=w432) -> (timed out?=w427:bool, error out=w428:errorcluster)  [unwired: 1 out]
        n195 = case shown="True" w427 {
          tunnel: w430 -> [_ w443]
          tunnel: w429 -> [_ w442]
          tunnel: w428 -> [w435 w441]
          tunnel: [w435 w438] -> w426
          frame False {
          }
          frame True {
            w436 = 500  # Prevent core stuck, but cause loosing command
            n196 = Enqueue Element At Opposite End(queue=w443, element=w442, timeout in ms (-1)=w436, error in (no error)=w441) -> (queue out=w440:refnum<queue>, error out=w437:errorcluster)  [unwired: 1 out]
            n197 = Enqueue Element At Opposite End(queue=w440, element=T4 {"State"=enum."UpdateXPos", "Params."=variant}, timeout in ms (-1)=w436, error in (no error)=w437) -> (error out=w438:errorcluster)  [unwired: 2 out]
          }
        }
      }
      frame "GetVelocity", "GetAcceleration" {
        # "system does not response \nafter a command is received"
        # "timeout push command back then do update?\n\npreventing blocking"
        n198 = Enqueue Element(queue=w450, element=w448, error in (no error)=w449) -> (queue out=w445:refnum<queue>, error out=w444:errorcluster)  [unwired: 1 in, 1 out]
        n199 = Enqueue Element(queue=w445, element=T4 {"State"=enum."_SettingReturn", "Params."=variant}, error in (no error)=w444) -> (error out=w447:errorcluster)  [unwired: 1 in, 2 out]
      }
      frame "_SettingReturn" {
        n200 = Unbundle By Name(w460) -> ("Params."=w459:variant)
        n201 = Variant To Data(error in=w453, type=cluster{"Acceleration":dbl[], "Velocity":dbl[]} {"Acceleration"=[], "Velocity"=[]}, Variant=w459) -> (data=w456:cluster{"Acceleration":dbl[], "Velocity":dbl[]}, error out=w452:errorcluster)
        n202 = Unbundle By Name(w456) -> ("Velocity"=w455:dbl[], "Acceleration"=w454:dbl[])
        n203 = Bundle By Name(cluster=w461, "Velocity"=w455, "Acceleration"=w454) -> (w458:T5)
      }
      frame "JoyStick" {
        n204 = Unbundle By Name(w473) -> ("Params."=w472:variant)
        n205 = Preview Queue Element(queue=w468) -> (queue out=w463:refnum<queue>, element=w466:T4)  [unwired: 2 in, 2 out]
        n206 = Unbundle By Name(w466) -> ("State"=w465:T1)
        n207 = Variant To Data(type=cluster{"Axis":i32, "Speed(rev/s)":dbl} {"Axis"=0, "Speed(rev/s)"=0.0}, Variant=w472) -> (data=w470:cluster{"Axis":i32, "Speed(rev/s)":dbl}, error out=w467:errorcluster)  [unwired: 1 in]
        n208 = Equal?(x=w465, y=T8."JoyStick" ("State")) -> ()  [unwired: 1 out]
        n209 = Or(x=w467, y=FALSE ("status")) -> (x .or. y?=w469:bool)
        n210 = Unbundle By Name(w475) -> ("CommPort"=w474:refnum<visa-resource-name>)
        n211 = case shown="False" w469 {
          tunnel: [w488 w489] -> w476
          tunnel: w474 -> [w486 _]
          tunnel: w470 -> [w485 _]
          tunnel: w467 -> [w481 w489]
          tunnel: w463 -> [w480 _]
          frame False {
            # "update after joystick move"
            n212 = Unbundle By Name(w485) -> ("Speed(rev/s)"=w478:dbl, "Axis"=w477:i32)
            n213 = Enqueue Element At Opposite End(queue=w480, element=T4 {"State"=enum."UpdateAll", "Params."=variant}) -> ()  [unwired: 2 in, 3 out]
            n214 = Format Into String(format string="%f %d speed", error in=w481, w478, w477) -> (resulting string=w484:string, error out=w483:errorcluster)  [unwired: 1 in]
            n215 = call <instrlib>:"VISA_Write+Read.vi"("Read? (T)"=FALSE ("Read?"), "error in (no error)"=w483, "Write Buffer"=w484, "VISA resource name"=w486) -> ("error out"=w488:errorcluster)  [unwired: 5 in, 2 out]
          }
          frame True {
          }
        }
      }
    }
    n216 = feedback #3() -> (w205:i32)
    n217 = Add(x=w205, y=w207) -> (x+y=w206:i32)
    "resfresh counter" <- w206
    n218 = feedback-in #3(w206) -> ()
    n219 = call <userlib>:"ErrorLog.vi"("error in (no error)"=w204) -> ("error out"=w203:errorcluster)  [unwired: 10 in]
  }
  n220 = while {
    tunnel: w15 -> [w503]
    shift-right: [w495] -> w6
    shift-left: w43 -> [w498]
    shift-right: [w500] -> _
    shift-left: refnum<visa-resource-name> refnum ("CommPort") -> [w504]
    shift-right: [w510] -> _
    shift-left: _ -> [w509]
    shift-right: [w506] -> _
    shift-left: FALSE -> [w507]
    tunnel: w17 -> [w494]
    shift-right: [w493] -> _
    shift-left: cluster{"Acceleration":dbl[], "Velocity":dbl[]} {"Acceleration"=[], "Velocity"=[]} -> [w492]
    i -> [w490]
    stop <- w513 stop-if-true
    # "Blocking Comand Loop"
    n221 = Dequeue Element(queue=w503) -> (queue out=w491:refnum<queue>, element=w505:T4, error out=w512:errorcluster)  [unwired: 2 in, 1 out]
    n222 = Unbundle By Name(w505) -> ("Params."=w508:variant, "State"=w511:T1)
    "State(Blocking)" <- w511
    n223 = Merge Errors(w512, w498) -> (w502:errorcluster)
    n224 = case shown="\"MoveAbs_all\"" w511 {
      tunnel: w505 -> [w527 _ _ _ _ _ _ _ _ _ _ _ _ _ _ _ _ _ _ _ _ w723]
      tunnel: [_ _ _ TRUE _ _ _ _ _ _ _ _ _ _ _ _ _ _ _ _ _ _] -> w513
      tunnel: [w524 w531 w542 w553 w559 w572 w583 w593 w605 w609 w626 w638 errorcluster {"status"=FALSE, "code"=0, "source"=""} ("error out") w653 w662 w667 w678 w686 w690 w702 w711 w726] -> w497
      tunnel: w502 -> [w525 w532 w543 w553 w560 w569 w576 w590 w598 w616 w628 w640 _ w653 w661 w668 w676 w686 w698 w708 w710 w726]
      tunnel: [w520 w530 refnum<visa-resource-name> refnum ("CommPort") w552 w558 w571 w581 w592 w603 w615 w630 w642 w647 w652 w657 w665 w674 w685 w697 w707 w718 w727] -> w500
      tunnel: w504 -> [_ w530 w544 w552 w558 w571 w581 w592 w603 w615 w630 w642 w647 w652 w657 w665 w675 w685 w697 w707 w718 w727]
      tunnel: w491 -> [_ _ _ _ _ _ _ _ _ _ _ _ _ _ _ _ _ _ _ _ _ _]
      tunnel: [w521 w533 w540 w551 w562 w574 w582 w595 w604 w618 w631 w643 w646 w651 w658 w666 w680 w684 w696 w706 w717 w725] -> w510
      tunnel: w509 -> [_ w533 w540 w551 w562 w574 w582 w595 w604 w618 w631 w643 w646 w651 w658 w666 w680 w684 w696 w706 w717 w725]
      tunnel: w508 -> [_ _ _ _ _ w570 w579 w591 w601 w614 w629 w641 _ _ w659 w669 _ _ _ _ _ _]
      tunnel: w507 -> [_ w529 w539 w550 w561 w573 w580 w594 w602 w617 w625 w637 w645 w650 w663 w673 w681 w683 w699 w709 w716 w724]
      tunnel: [w519 w529 w539 w550 w561 w573 w580 w594 w602 w617 w625 w637 w645 w650 w663 w673 w681 w683 w699 w709 w716 w724] -> w506
      tunnel: w494 -> [_ _ _ _ _ _ _ _ _ _ _ _ _ _ _ _ _ _ _ _ w715 _]
      tunnel: [w518 w528 w538 w549 w555 w563 w575 w584 w596 w608 w621 w633 w644 w649 w654 w664 w679 w682 w695 w705 w712 w719] -> w493
      tunnel: w492 -> [w518 w528 w538 w549 w555 w563 w575 w584 w596 w608 w621 w633 w644 w649 w654 w664 w679 w682 w694 w701 w712 w719]
      frame "Initialize" {
        # "open port, set default config"
        n225 = Unbundle By Name(w527) -> ("Params."=w526:variant)
        n226 = Variant To Data(error in=w525, type=T5 {"Position"=[], "Velocity"=[], "Acceleration"=[], "Moving"=FALSE, "Simulation"=FALSE, "tickcount_mov"=0, "tickcount_pos"=0, "NumOfAxis"=0, "Initialized"=FALSE, "CommPort"="", "Range"=[], "Serial Configuration"={"Baud Rate"=0, "Parity"=0, "Data Bits"=0, "Stop Bits"=0, "Flow Control"=0}, "MotorDisabled"=refnum}, Variant=w526) -> (data=w522:T5, error out=w524:errorcluster)
        n227 = Unbundle By Name(w522) -> ("Simulation"=w519:bool, "NumOfAxis"=w521:i32, "CommPort"=w520:refnum<visa-resource-name>)
      }
      frame "SetDefaultConfig" {
        # "Not need for this"
        n228 = case shown="False" w529 {
          tunnel: w532 -> [w536 w537]
          tunnel: [w535 w537] -> w531
          tunnel: w530 -> [w534 _]
          frame False {
            n229 = call <instrlib>:"Default Instrument Setup.vi"("error in (no error)"=w536, "VISA resource name"=w534) -> ("error out"=w535:errorcluster)  [unwired: 8 in, 1 out]
          }
          frame True {
          }
        }
      }
      frame "Close" {
        n230 = case shown="True" w539 {
          tunnel: w544 -> [_ w548]
          tunnel: w543 -> [w545 w547]
          tunnel: [w545 w546] -> w542
          frame False {
          }
          frame True {
            n231 = VISA Close(VISA resource name=w548, error in (no error)=w547) -> (error out=w546:errorcluster)
          }
        }
      }
      frame "Quit" {
      }
      frame "Identify" {
        n232 = call <instrlib>:"Revision Query.vi"("error in (no error)"=w560, "VISA resource name"=w558) -> ("error out"=w559:errorcluster, "Instrument Firmware Revision"=→"Instrument Firmware Revision":string, "Instrument Driver Revision"=→"Instrument Driver Revision":string)  [unwired: 6 in, 1 out]
      }
      frame "MoveAbs" {
        n233 = Variant To Data(error in=w569, type=cluster{"Axis":i32, "Position":dbl} {"Axis"=0, "Position"=0.0}, Variant=w570) -> (data=w566:cluster{"Axis":i32, "Position":dbl}, error out=w568:errorcluster)
        n234 = Unbundle By Name(w566) -> ("Position"=w564:dbl, "Axis"=w565:i32)
        n235 = call <instrlib>:"MoveAbs.vi"("error in"=w568, "Axis"=w565, "Position"=w564, "VISA resource"=w571) -> ("error out"=w572:errorcluster)  [unwired: 7 in]
      }
      frame "MoveAbs_all" {
        n236 = Variant To Data(error in=w576, type=dbl[] [] ("Position"), Variant=w579) -> (data=w578:dbl[])  [unwired: 1 out]
        n237 = call <instrlib>:"MoveAbs_all.vi"("# axis"=w582, "Position"=w578, "VISA resource name"=w581) -> ("error out"=w583:errorcluster)  [unwired: 8 in]
      }
      frame "MoveRel" {
        n238 = Variant To Data(error in=w590, type=cluster{"Axis":i32, "Distance":dbl} {"Axis"=0, "Distance"=0.0}, Variant=w591) -> (data=w587:cluster{"Axis":i32, "Distance":dbl}, error out=w589:errorcluster)
        n239 = Unbundle By Name(w587) -> ("Distance"=w585:dbl, "Axis"=w586:i32)
        n240 = call <instrlib>:"MoveRef.vi"("error in"=w589, "Axis"=w586, "Position"=w585, "VISA resource"=w592) -> ("error out"=w593:errorcluster)  [unwired: 7 in]
      }
      frame "MoveRel_all" {
        # "axis# in parameter can surpass\nactual axis#, excess axis will not\ndiscard"
        n241 = Variant To Data(error in=w598, type=dbl[] [] ("Position"), Variant=w601) -> (data=w600:dbl[], error out=w597:errorcluster)
        n242 = call <instrlib>:"MoveRel_all.vi"("# axis"=w604, "error in (no error)"=w597, "Position"=w600, "VISA resource name"=w603) -> ("error out"=w605:errorcluster)  [unwired: 7 in]
      }
      frame "WaitStop" {
        n243 = call <instrlib>:"WaitStop.vi"("error in (no error)"=w616, "VISA resource name"=w615) -> ("error out"=w609:errorcluster, "Com failure Counts"=→"Com failure#":i32)  [unwired: 7 in, 1 out]
        n244 = Variant To Data(type=refnum<queue> refnum ("Feedback"), Variant=w614) -> (data=w612:refnum<queue>)  [unwired: 1 in, 1 out]
        n245 = call <vilib>:"Clear Errors.vi"("error in (no error)"=w609) -> ("error out"=w607:errorcluster)  [unwired: 5 in, 1 out]
        n246 = Enqueue Element(queue=w612, element="Done", error in (no error)=w607) -> (error out=w610:errorcluster)  [unwired: 1 in, 2 out]
        n247 = call <vilib>:"Clear Errors.vi"("error in (no error)"=w610) -> ()  [unwired: 5 in, 2 out]
      }
      frame "SetVelocity" {
        n248 = Variant To Data(error in=w628, type=cluster{"Axis":i32, "Velocity":dbl} {"Axis"=0, "Velocity"=0.0}, Variant=w629) -> (data=w623:cluster{"Axis":i32, "Velocity":dbl}, error out=w627:errorcluster)
        n249 = Unbundle By Name(w623) -> ("Velocity"=w622:dbl)
        n250 = Multiply(x=w622, y=60.0) -> (x*y=w620:dbl)
        n251 = call <instrlib>:"SetVelocity.vi"("error in"=w627, "Velocity"=w620, "VISA resource"=w630) -> ("error out"=w626:errorcluster)  [unwired: 8 in]
      }
      frame "SetAcceleration" {
        n252 = Variant To Data(error in=w640, type=cluster{"Axis":i32, "Acceleration":dbl} {"Axis"=0, "Acceleration"=0.0}, Variant=w641) -> (data=w635:cluster{"Axis":i32, "Acceleration":dbl}, error out=w639:errorcluster)
        n253 = Unbundle By Name(w635) -> ("Axis"=w632:i32, "Acceleration"=w634:dbl)
        n254 = call <instrlib>:"SetAcceleration.vi"("error in"=w639, "Acceleration"=w634, "Axial #"=w632, "VISA resource"=w642) -> ("error out"=w638:errorcluster)  [unwired: 7 in]
      }
      frame "ClearErr" {
      }
      frame "LogMessage" {
      }
      frame "MotorEnable(1)" {
        n255 = Variant To Data(error in=w661, type=FALSE ("On/Off"), Variant=w659) -> (data=w655:bool, error out=w660:errorcluster)
        n256 = call <instrlib>:"MotorOnOff.vi"("#Axis"=w658, "error in"=w660, "Enabled"=w655, "VISA resource"=w657) -> ("error out"=w662:errorcluster)  [unwired: 7 in]
      }
      frame "EnableAxis" {
        # "This can be done better"
        n257 = Variant To Data(error in=w668, type=FALSE ("On/Off"), Variant=w669) -> (data=w670:bool, error out=w672:errorcluster)
        n258 = call <instrlib>:"MotorOnOff.vi"("#Axis"=w666, "error in"=w672, "Enabled"=w670, "VISA resource"=w665) -> ("error out"=w667:errorcluster)  [unwired: 7 in]
      }
      frame "SoftReset" {
        n259 = call <vilib>:"Clear Errors.vi"("error in (no error)"=w676) -> ("error out"=w677:errorcluster)  [unwired: 5 in, 1 out]
        n260 = call <instrlib>:"Reset.vi"("error in (no error)"=w677, "VISA resource name"=w675) -> ("error out"=w678:errorcluster, "VISA resource name out"=w674:refnum<visa-resource-name>)  [unwired: 8 in]
      }
      frame "JoyStick" {
      }
      frame "GetVelocity" {
        n261 = Unbundle By Name(w694) -> ("Velocity"=w692:dbl[])
        n262 = call <instrlib>:"GetVelocity.vi"("error in (no error)"=w698, "VISA resource name"=w697) -> ("error out"=w690:errorcluster, "Velocity"=w689:dbl)  [unwired: 8 in]
        n263 = Divide(x=w689, y=60.0) -> (x/y=w688:dbl)
        n264 = Initialize Array(w688, w696) -> (w691:dbl[])
        n265 = Select(t=w692, s=w690, f=w691) -> (s? t:f=w693:dbl[])
        n266 = Bundle By Name(cluster=w694, "Velocity"=w693) -> (w695:cluster{"Acceleration":dbl[], "Velocity":dbl[]})
      }
      frame "GetAcceleration" {
        n267 = Unbundle By Name(w701) -> ("Acceleration"=w703:dbl[])
        n268 = call <instrlib>:"GetAcceleration.vi"("error in (no error)"=w708, "VISA resource name"=w707) -> ("error out"=w702:errorcluster, "Acceleration"=w700:dbl[])  [unwired: 8 in]
        n269 = Select(t=w703, s=w702, f=w700) -> (s? t:f=w704:dbl[])
        n270 = Bundle By Name(cluster=w701, "Acceleration"=w704) -> (w705:cluster{"Acceleration":dbl[], "Velocity":dbl[]})
      }
      frame "_SettingReturn" {
        n271 = Bundle By Name(cluster=T4 {"State"=enum."_SettingReturn", "Params."=variant} ("element"), "Params."=w712) -> (w713:T4)
        n272 = Enqueue Element(queue=w715, element=w713, error in (no error)=w710) -> (error out=w711:errorcluster)  [unwired: 1 in, 2 out]
      }
      frame Default {
        n273 = Unbundle By Name(w723) -> ("State"=w721:T1)
        n274 = Format Into String(format string="\nUnsupported command:%d,\nDefault frame", w721) -> (resulting string=w722:string)  [unwired: 2 in, 1 out]
        n275 = One Button Dialog(message=w722) -> ()  [unwired: 1 in, 1 out]
      }
    }
    n276 = Equal?(x=w500, y=refnum<visa-resource-name> refnum ("CommPort")) -> (x = y?=w501:bool)
    n277 = case "Prevent FIFO jammed" shown="False" w501 {
      tunnel: w497 -> [w516 w517]
      tunnel: [w514 w517] -> w496
      tunnel: w500 -> [w515 _]
      frame False {
        n278 = call <instrlib>:"WaitStop.vi"("error in (no error)"=w516, "VISA resource name"=w515) -> ("error out"=w514:errorcluster)  [unwired: 7 in, 2 out]
      }
      frame True {
      }
    }
    n279 = call <userlib>:"ErrorLog.vi"("error in (no error)"=w496) -> ("error out"=w495:errorcluster)  [unwired: 10 in]
    "Blokcing Loop cts" <- w490
  }
  n280 = property class="Arr (strict)"(reference=w2, error in=w3, "Val(Sgnl)"=w4) -> ()  [unwired: 2 out]
  n281 = Merge Errors(w8, w6) -> (w14:errorcluster)
  "error out" <- w14
  n282 = Release Queue(queue=w15, error in (no error)=w14) -> ()  [unwired: 1 in, 3 out]
  n283 = Release Queue(queue=w16, error in (no error)=w14) -> ()  [unwired: 1 in, 3 out]
